vi "getStageFromXml.vi"(8 "error in (no error)":errorcluster, 10 "Xml":refnum<class "xmlNode.lvclass">, 11 "ScriptEvent in":refnum<class "ScriptEvent.lvclass">) -> (0 "error out":errorcluster, 2 "Xml out":refnum<class "xmlNode.lvclass">, 3 "ScriptEvent out":refnum<class "ScriptEvent.lvclass">)   [LabVIEW 2011, in "Tools.lvlib" / "Scripting.lvlib" / "ScriptEvent.lvclass"]
uses:
  ScriptEvent.lvclass
  xmlNode/xmlNode.lvclass
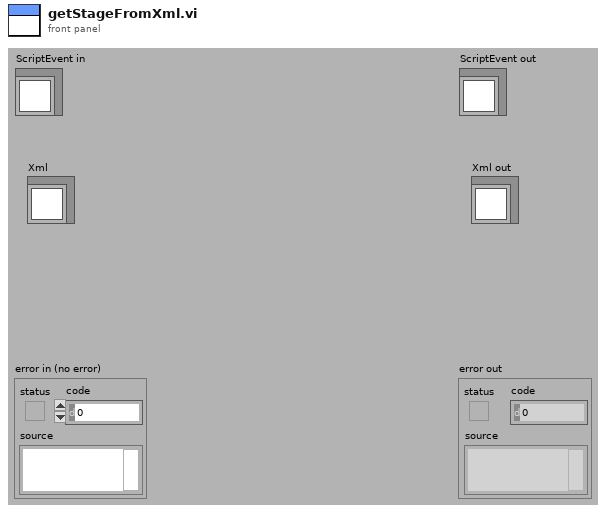
[diagram p1: front panel]
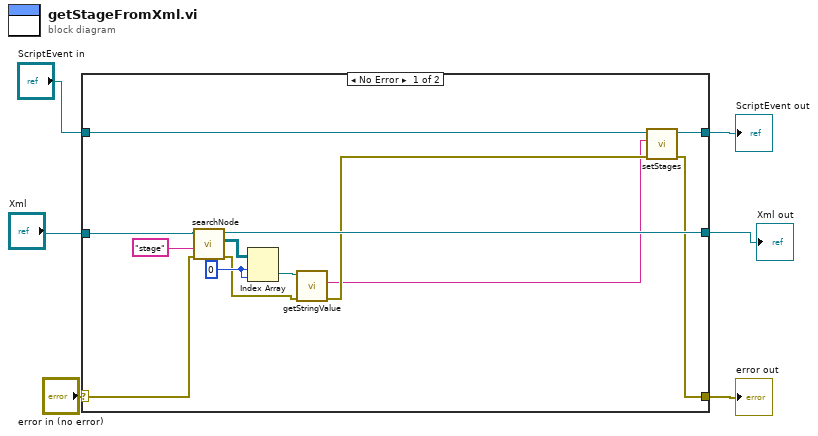
[diagram p0: block diagram]
diagram:
  n1 = case shown="No Error" "error in (no error)" {
    selector: "error in (no error)" -> [w13 w21]
    tunnel: [w8 w21] -> w5
    tunnel: [w11 w20] -> w3
    tunnel: "ScriptEvent in" -> [w10 w20]
    tunnel: "Xml" -> [w15 _]
    tunnel: [w14 _] -> w1
    frame No Error {
      w17 = 0
      n2 = call-dynamic "searchNode.vi"("error in (no error)"=w13, "searchElementName"="stage", "xmlNode in"=w15) -> ("error out"=w12:errorcluster, "arrayXmlNodes"=w18:refnum<class "xmlNode.lvclass">[][], "xmlNode out"=w14:refnum<class "xmlNode.lvclass">)  [unwired: 6 in]
      n3 = Index Array(array=w18, index (row)=w17, index (col)=w17) -> (element=w16:refnum<class "xmlNode.lvclass">)
      n4 = call-dynamic "getStringValue.vi"("error in (no error)"=w12, "xmlNode.lvclass in"=w16) -> ("error out"=w9:errorcluster, "stringValue"=w7:string)  [unwired: 7 in, 1 out]
      n5 = call-dynamic "setStages.vi"("error in (no error)"=w9, "Stage"=w7, "ScriptEvent.lvclass in"=w10) -> ("error out"=w8:errorcluster, "ScriptEvent.lvclass out"=w11:refnum<class "ScriptEvent.lvclass">)  [unwired: 7 in]
    }
    frame Error {
    }
  }
  "error out" <- w5
  "ScriptEvent out" <- w3
  "Xml out" <- w1
